vi "Abort.vi"(8 "error in (no error)":errorcluster, 11 "Process Events":T1) -> (0 "error out":errorcluster, 3 "Process Events out":T1)   [LabVIEW 2015, in "Simple Progress Bar.lvlib"]
uses:
  Simple Progress Bar.lvlib
  Process Events.ctl
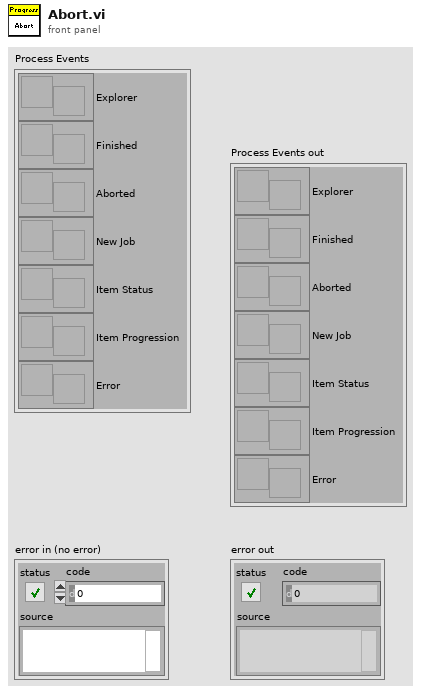
[diagram p1: front panel]
types:
  T1 = typedef "Simple Progress Bar.lvlib/Process Events.ctl" = cluster{"Explorer":refnum<user-event>, "Finished":refnum<user-event>, "Aborted":refnum<user-event>, "New Job":refnum<user-event>, "Item Status":refnum<user-event>, "Item Progression":refnum<user-event>, "Error":refnum<user-event>}
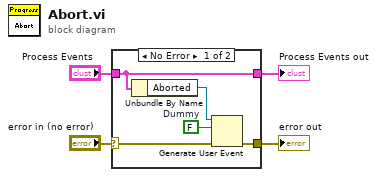
[diagram p0: block diagram]
diagram:
  n1 = case shown="No Error" "error in (no error)" {
    selector: "error in (no error)" -> [w7 w10]
    tunnel: "Process Events" -> [w5 w11]
    tunnel: [w5 w11] -> w2
    tunnel: [w6 w10] -> w1
    frame No Error {
      w8 = FALSE  # Dummy
      n2 = Unbundle By Name(w5) -> ("Aborted"=w9:refnum<user-event>)
      n3 = Generate User Event(user event=w9, event data cluster=w8, error in=w7) -> (error out=w6:errorcluster)  [unwired: 1 in, 1 out]
    }
    frame Error {
    }
  }
  "error out" <- w1
  "Process Events out" <- w2
